vi "Info File.vi"(8 "Run Folder path":path) -> ()   [LabVIEW 2015]
uses:
  Global for Tr-ARPES.vi
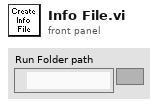
[diagram p1: front panel]
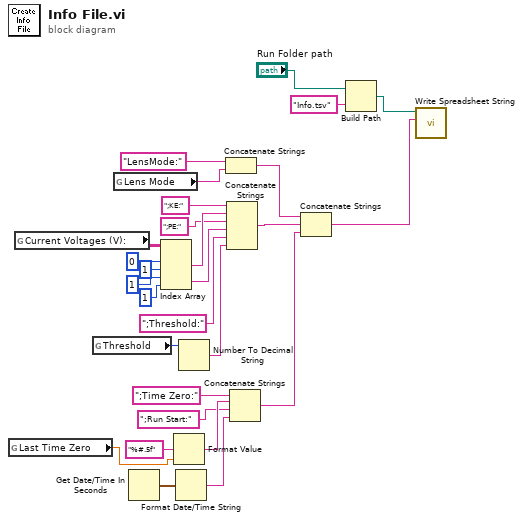
[diagram p0: block diagram]
diagram:
  n1 = global read "Global for Tr-ARPES.vi" "Last Time Zero"() -> (w13:dbl)
  n2 = global read "Global for Tr-ARPES.vi" "Current Voltages (V):"() -> (w18:string[][])
  n3 = global read "Global for Tr-ARPES.vi" "Threshold"() -> (w4:u32)
  n4 = global read "Global for Tr-ARPES.vi" "Lens Mode"() -> (w24:string)
  n5 = Get Date/Time In Seconds() -> (seconds since 1Jan1904=w10:timestamp)
  n6 = Index Array(array=w18, index (row) #1=0 ("disabled index (row)"), index (col) #1=1 ("disabled index (col)"), index (row) #2=1 ("disabled index (row)"), index (col) #2=1 ("index (col)")) -> (element #1=w17:string, element #2=w15:string)
  n7 = Format Value(format string="%#.5f", value (0)=w13) -> (output string=w11:string)  [unwired: 1 in]
  n8 = Format Date/Time String(seconds (now)=w10) -> (date/time string=w9:string)  [unwired: 2 in]
  n9 = Number To Decimal String(number=w4) -> (decimal integer string=w1:string)  [unwired: 1 in]
  n10 = Concatenate Strings("LensMode:" ("string"), w24) -> (w6:string)
  n11 = Concatenate Strings(";KE:" ("string"), w17, ";PE:" ("string"), w15, ";Threshold:" ("string"), w1) -> (w8:string)
  n12 = Concatenate Strings(";Time Zero:" ("string"), w11, ";Run Start:" ("string"), w9) -> (w7:string)
  n13 = Concatenate Strings(w6, w8, w7) -> (w5:string)
  n14 = Build Path(base path="Run Folder path", name or relative path="Info.tsv") -> (appended path=w27:path)
  n15 = call <vilib>:"Write Spreadsheet String.vi"("spreadsheet string"=w5, "file path (dialog if empty)"=w27) -> ()  [unwired: 8 in, 2 out]
